vi "Valid.vi"(11 "Send in":refnum<class "Send.lvclass">) -> (2 "Valid?":bool, 3 "Send out":refnum<class "Send.lvclass">)   [LabVIEW 2011, in "Messenging.lvlib" / "Send.lvclass"]
uses:
  Send.lvclass
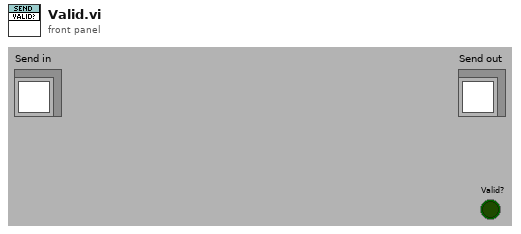
[diagram p1: front panel]
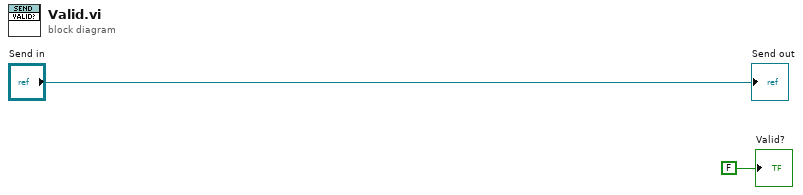
[diagram p0: block diagram]
diagram:
  "Send out" <- "Send in"
  "Valid?" <- FALSE ("Valid?")
